vi "Wait on Boolean.vi"(8 "error in (no error)":errorcluster, 11 "Global boolean to wait on":T1) -> (0 "error out":errorcluster)   [LabVIEW 2014]
uses:
  Global Booleans Enum.ctl
  Globals.vi
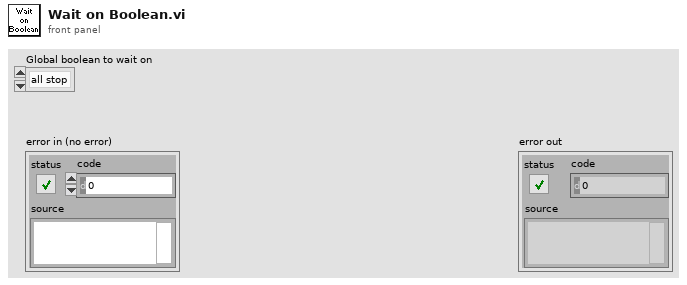
[diagram p1: front panel]
types:
  T1 = typedef "Global Booleans Enum.ctl" = enum16{"all stop", "Play", "Image Aligned?"}
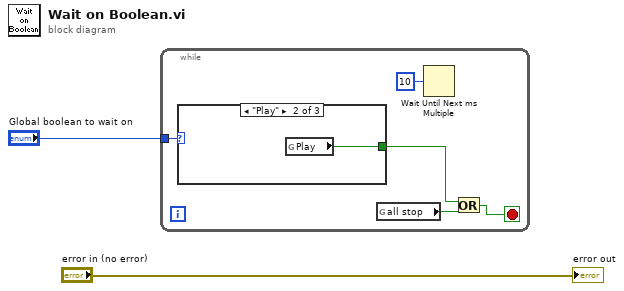
[diagram p0: block diagram]
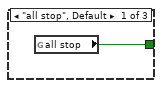
[diagram p2: hidden frame]
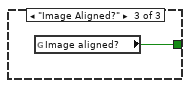
[diagram p3: hidden frame]
diagram:
  n1 = while {
    tunnel: "Global boolean to wait on" -> [w4]
    stop <- w6 stop-if-true
    n2 = case shown="\"Play\"" w4 {
      tunnel: [w8 w9 w10] -> w3
      frame "all stop", Default {
        n3 = global read "Globals.vi" "all stop"() -> (w8:bool)
      }
      frame "Play" {
        n4 = global read "Globals.vi" "Play"() -> (w9:bool)
      }
      frame "Image Aligned?" {
        n5 = global read "Globals.vi" "Image aligned?"() -> (w10:bool)
      }
    }
    n6 = global read "Globals.vi" "all stop"() -> (w7:bool)
    n7 = Wait Until Next ms Multiple(millisecond multiple=u32 10) -> ()  [unwired: 1 out]
    n8 = Or(x=w3, y=w7) -> (x .or. y?=w6:bool)
  }
  "error out" <- "error in (no error)"
